vi "Wash Steps Selected.vi"(8 "error in (no error)":errorcluster, 11 "Wash Options Ref":refnum<vi>) -> (0 "error out":errorcluster, 1 "Wash Steps Selected-Update Display Message":T1)   [LabVIEW 2020]
doc: "This VI reads the Wash Options menu and creates an array with the selected options."
uses:
  Controls/Wash Steps Selected-Update Display Message.ctl
  Controls/Wash Steps Selected.ctl
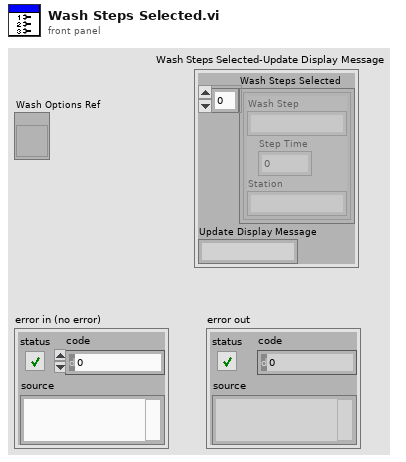
[diagram p1: front panel]
types:
  T1 = typedef "Wash Steps Selected-Update Display Message.ctl" = cluster{"Wash Steps Selected":cluster{"Wash Step":string, "Step Time":i32, "Station":string}[], "Update Display Message":string}
  T2 = enum8{"Enabled", "Disabled", "Disabled and Grayed Out"}
  T3 = cluster{bool, bool, bool, bool, bool, bool, bool, bool}
  T4 = typedef "Wash Steps Selected.ctl" = cluster{"Wash Step":string, "Step Time":i32, "Station":string}[]
  T5 = cluster{"Wash Step":string, "Step Time":i32, "Station":string}[]
  T6 = cluster{"Wash Step":string, "Step Time":i32, "Station":string}
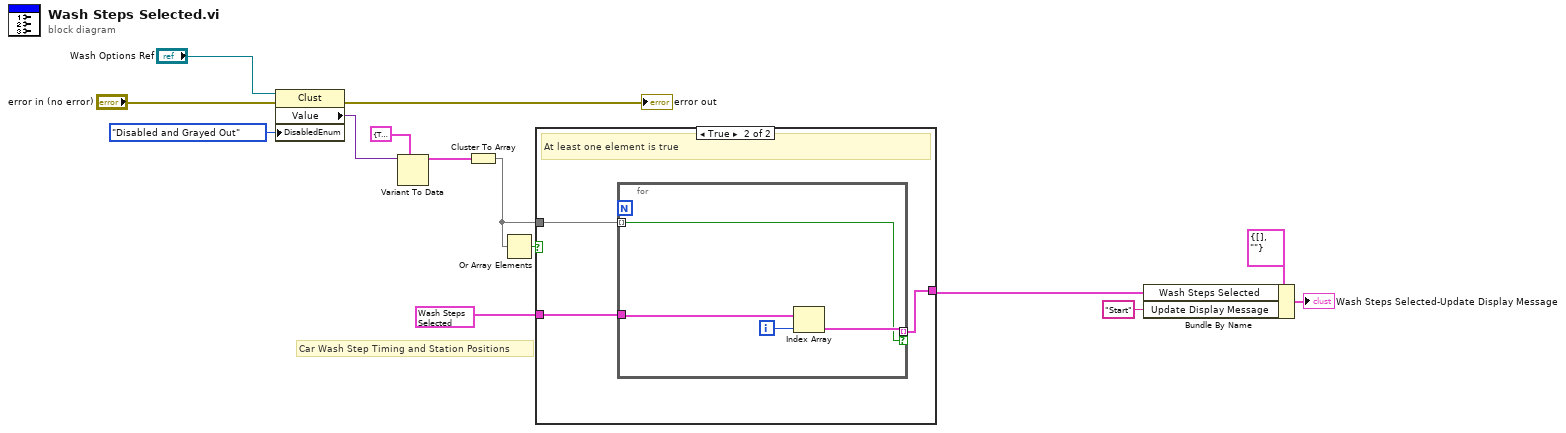
[diagram p0: block diagram]
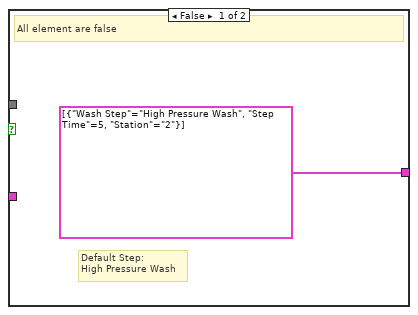
[diagram p2: hidden frame]
diagram:
  # "Car Wash Step Timing and Station Positions"
  n1 = property class="Clust"(reference="Wash Options Ref", error in="error in (no error)", "DisabledEnum"=T2."Disabled and Grayed Out" ("Disabled")) -> (error out=→"error out":errorcluster, "Value"=w11:variant)  [unwired: 1 out]
  n2 = Variant To Data(type=T3 {TRUE, TRUE, TRUE, TRUE, TRUE, TRUE, TRUE, TRUE}, Variant=w11) -> (data=w9:T3)  [unwired: 1 in, 1 out]
  n3 = Cluster To Array(cluster=w9) -> (array=w6:bool[])
  n4 = Or Array Elements(Boolean array=w6) -> (logical OR=w8:bool)
  n5 = case shown="True" w8 {
    tunnel: T4 [{"Wash Step"="Under Body Wash", "Step Time"=5, "Station"="1"}, {"Wash Step"="Bug Remover", "Step Time"=5, "Station"="1"}, {"Wash Step"="Pre-Soak", "Step Time"=5, "Station"="2"}, {"Wash Step"="High Pressure Wash", "Step Time"=5, "Station"="2"}, {"Wash Step"="Low Pressure Wax", "Step Time"=5, "Station"="2"}, {"Wash Step"="Spot Free Rinse", "Step Time"=5, "Station"="2"}, {"Wash Step"="Tire Shine Foam", "Step Time"=5, "Station"="3"}, {"Wash Step"="Air Dry", "Step Time"=5, "Station"="3"}] -> [_ w17]
    tunnel: [T5 [{"Wash Step"="High Pressure Wash", "Step Time"=5, "Station"="2"}] w16] -> w4
    tunnel: w6 -> [_ w18]
    frame False {
      # "Default Step:\nHigh Pressure Wash"
      # "All element are false"
    }
    frame True {
      # "At least one element is true"
      n6 = for {
        tunnel: w18 -> [w19] mode=indexing
        tunnel: w17 -> [w22]
        tunnel: [w20] -> w16 mode=indexing if=w19
        i -> [w21]
        n7 = Index Array(array=w22, index=w21) -> (element=w20:T6)
      }
    }
  }
  n8 = Bundle By Name(cluster=T1 {"Wash Steps Selected"=[], "Update Display Message"=""}, "Wash Steps Selected"=w4, "Update Display Message"="Start") -> (→"Wash Steps Selected-Update Display Message":T1)
